vi "OEE_SCREEN_1_recolor_quality_yeild.vi"(1 "quality_yeild_field_reference":refnum<vi>, 2 "quality_yeild_value":string) -> ()   [LabVIEW 2019]
uses:
  FGV/SQL_raw_data/FGV_OEE_SQL_raw_data.ctl
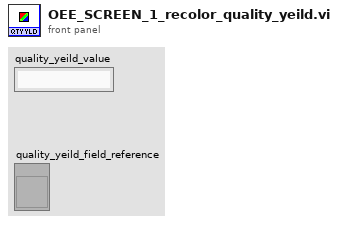
[diagram p1: front panel]
types:
  T1 = typedef "FGV_OEE_SQL_raw_data.ctl" = enum16{"initialize", "set_reference_name", "set_timestamp", "set_OK_NOK_count", "set_config_info", "set_pace", "set_availability", "set_hourly_ok_count", "set_targets", "get_all_info"}
  T2 = typedef "OEE_SQL_raw_data.ctl" = cluster{"reference_name":string, "data_timestamp":timestamp, "OK_NOK_count":string[][], "config_info":string[], "pace":string[][], "availability":string[], "hourly_ok_count":string[][], "shift_number":i8, "shift_start":i8, "shift_end":i8, "TAKT":u16, "FTTH_target":u16, "BOTTLENECK_station":string, "targets_hourly":u16[], "target_shift":u16}
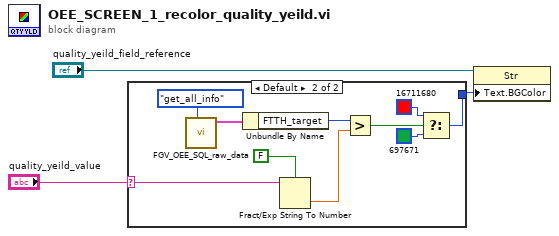
[diagram p0: block diagram]
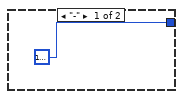
[diagram p2: hidden frame]
diagram:
  n1 = case shown="Default" "quality_yeild_value" {
    selector: "quality_yeild_value" -> [_ w7]
    tunnel: [u32 16777222 w14] -> w3
    frame "-" {
    }
    frame Default {
      n2 = call "FGV_OEE_SQL_raw_data.vi"("options"=FGV_OEE_SQL_raw_data."get_all_info") -> ("SQL_raw_data_out"=w6:T2)  [unwired: 9 in, 1 out]
      n3 = Unbundle By Name(w6) -> ("FTTH_target"=w9:u16)
      n4 = Fract/Exp String To Number(use system decimal point (T)=FALSE, string=w7) -> (number=w10:dbl)  [unwired: 2 in, 1 out]
      n5 = Greater?(x=w9, y=w10) -> (0:w12:bool)
      n6 = Select(t=u32 16711680, s=w12, f=u32 697671) -> (s? t:f=w14:u32)
    }
  }
  n7 = property class="Str"(reference="quality_yeild_field_reference", "Text.BGColor"=w3) -> ()  [unwired: 1 in, 2 out]
